vi "NameMap-Store.vi"(8 "error in (no error)":errorcluster, 10 "name":string, 11 "NameMap in":T1) -> (0 "error out":errorcluster, 3 "NameMap out":T1)   [LabVIEW 2019, in "lv-apt-json-file.lvlib"]
uses:
  lv-apt-json-file.lvlib
  Typedef/Def-NameMap.ctl
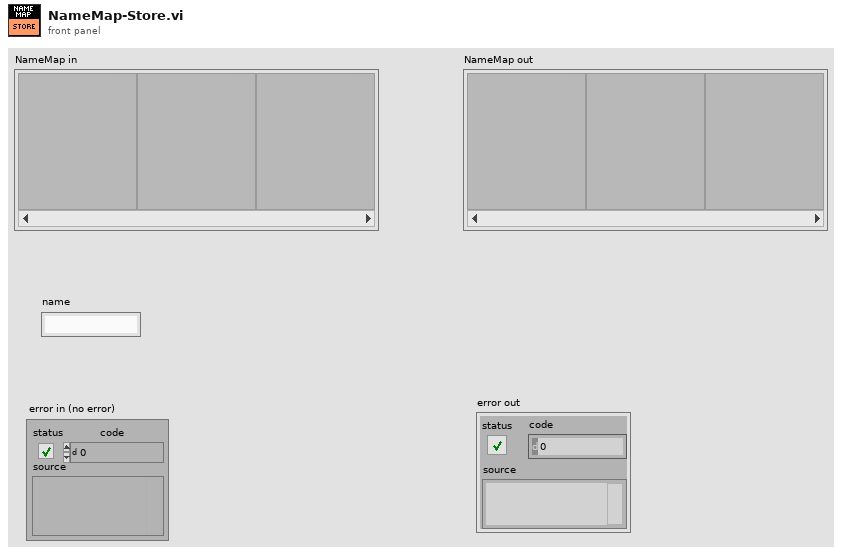
[diagram p1: front panel]
types:
  T1 = typedef "lv-apt-json-file.lvlib/Def-NameMap.ctl" = variant[]
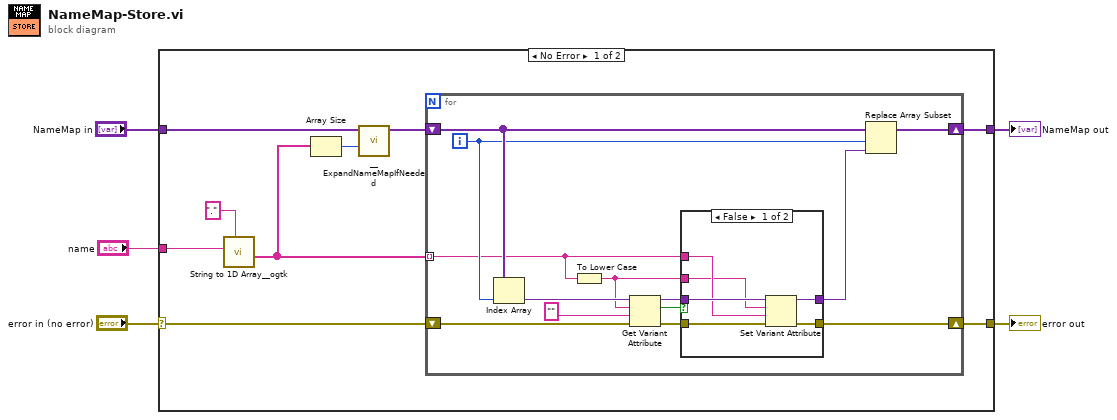
[diagram p0: block diagram]
diagram:
  n1 = case shown="No Error" "error in (no error)" {
    selector: "error in (no error)" -> [w11 w37]
    tunnel: "name" -> [w14 _]
    tunnel: [w12 w36] -> w4
    tunnel: [w10 w37] -> w2
    tunnel: "NameMap in" -> [w8 w36]
    frame No Error {
      n2 = call <userlib>:"String to 1D Array__ogtk.vi"("delimiter (Tab)"=".", "string"=w14) -> ("Array of Strings"=w9:string[])  [unwired: 9 in]
      n3 = Array Size(array=w9) -> (size(s)=w6:i32)
      n4 = call "__ExpandNameMapIfNeeded.vi"("Numeric"=w6, "NameMap A in"=w8) -> ("NameMap A out"=w7:T1)  [unwired: 9 in]
      n5 = for {
        shift-right: [w26] -> w12
        shift-left: w7 -> [w27]
        tunnel: w9 -> [w16] mode=indexing
        shift-right: [w20] -> w10
        shift-left: w11 -> [w19]
        i -> [w25]
        n6 = Index Array(array=w27, index=w25) -> (element=w24:variant)
        n7 = To Lower Case(string=w16) -> (all lower case string=w15:string)
        n8 = Get Variant Attribute(Variant=w24, name=w15, default value (empty Variant)="" ("delimiter (Tab)"), error in=w19) -> (duplicate Variant=w22:variant, found=w17:bool, error out=w21:errorcluster)  [unwired: 1 out]
        n9 = case shown="False" w17 {
          tunnel: w22 -> [w33 w35]
          tunnel: w16 -> [w29 _]
          tunnel: w21 -> [w32 w34]
          tunnel: [w31 w34] -> w20
          tunnel: [w30 w35] -> w18
          tunnel: w15 -> [w28 _]
          frame False {
            n10 = Set Variant Attribute(Variant=w33, name=w28, value=w29, error in=w32) -> (Variant out=w30:variant, error out=w31:errorcluster)  [unwired: 1 out]
          }
          frame True {
          }
        }
        n11 = Replace Array Subset(array=w27, new element=w18, index=w25) -> (w26:T1)
      }
    }
    frame Error {
    }
  }
  "NameMap out" <- w4
  "error out" <- w2
